vi "A170316-11_config.vi"() -> ()   [LabVIEW 2020]
uses:
  Global_Variable/Global.vi
  Database/Global1.vi
  <vilib>/Utility/config.llb/NI_LVConfig.lvlib
panel:
  in  "选项卡控件":enum32{"产品参数", "操作步骤", "产品管理"}(tab)
  in  "参数设定":string[][](table)
  in  "删除":bool
  in  "确定":bool
  in  "添加":bool
  in  "退出":bool
  in  "更新":bool
  in  "产品型号":string(combo)
  in  "安装电机操作步骤":T1
  in  "手柄安装步骤":T2
  in  "支架操作步骤":T3
  in  "请输入添加的产品名称":string
  in  "请选择要删除的产品":string(combo)
  # "调节机构装配"
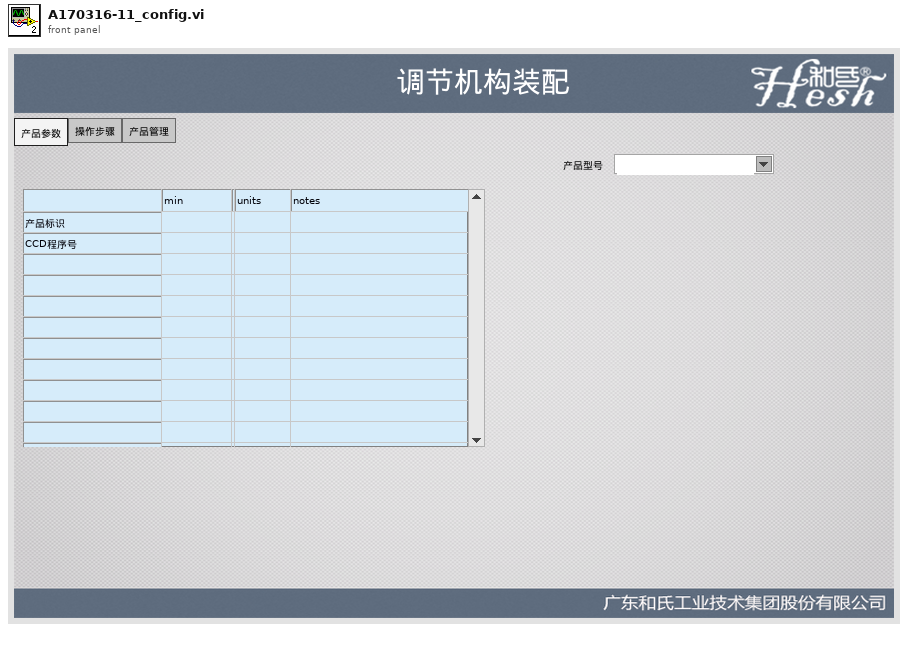
[diagram p1: front panel]
types:
  T1 = cluster{"安装弹簧":bool, "安装O型圈":bool, "安装弹性垫圈弹簧":bool, "电机安装螺栓1":bool, "电机安装螺栓2":bool, "电机安装螺栓3":bool, "电机拍照":bool, "涂色标":bool, "安装轧带":bool, "安装轧带取走工件":bool}
  T2 = cluster{"降噪垫片1/衬套1":bool, "降噪垫片2/衬套2":bool, "降噪块1":bool, "降噪块2":bool, "锁紧块":bool, "弹簧":bool, "滚针轴承":bool, "挡片":bool, "锁紧螺母":bool, "拍照":bool}
  T3 = cluster{"控制器支架螺栓1":bool, "控制器支架螺栓2":bool, "控制器支架螺栓3":bool, "控制器支架螺栓4":bool, "控制器支架螺栓5":bool, "控制器支架涂色标":bool, "控制器支架安装线束轧带":bool}
  T4 = typedef "NI_LVConfig.lvlib/Config Data RefNum.ctl" = refnum<k1>
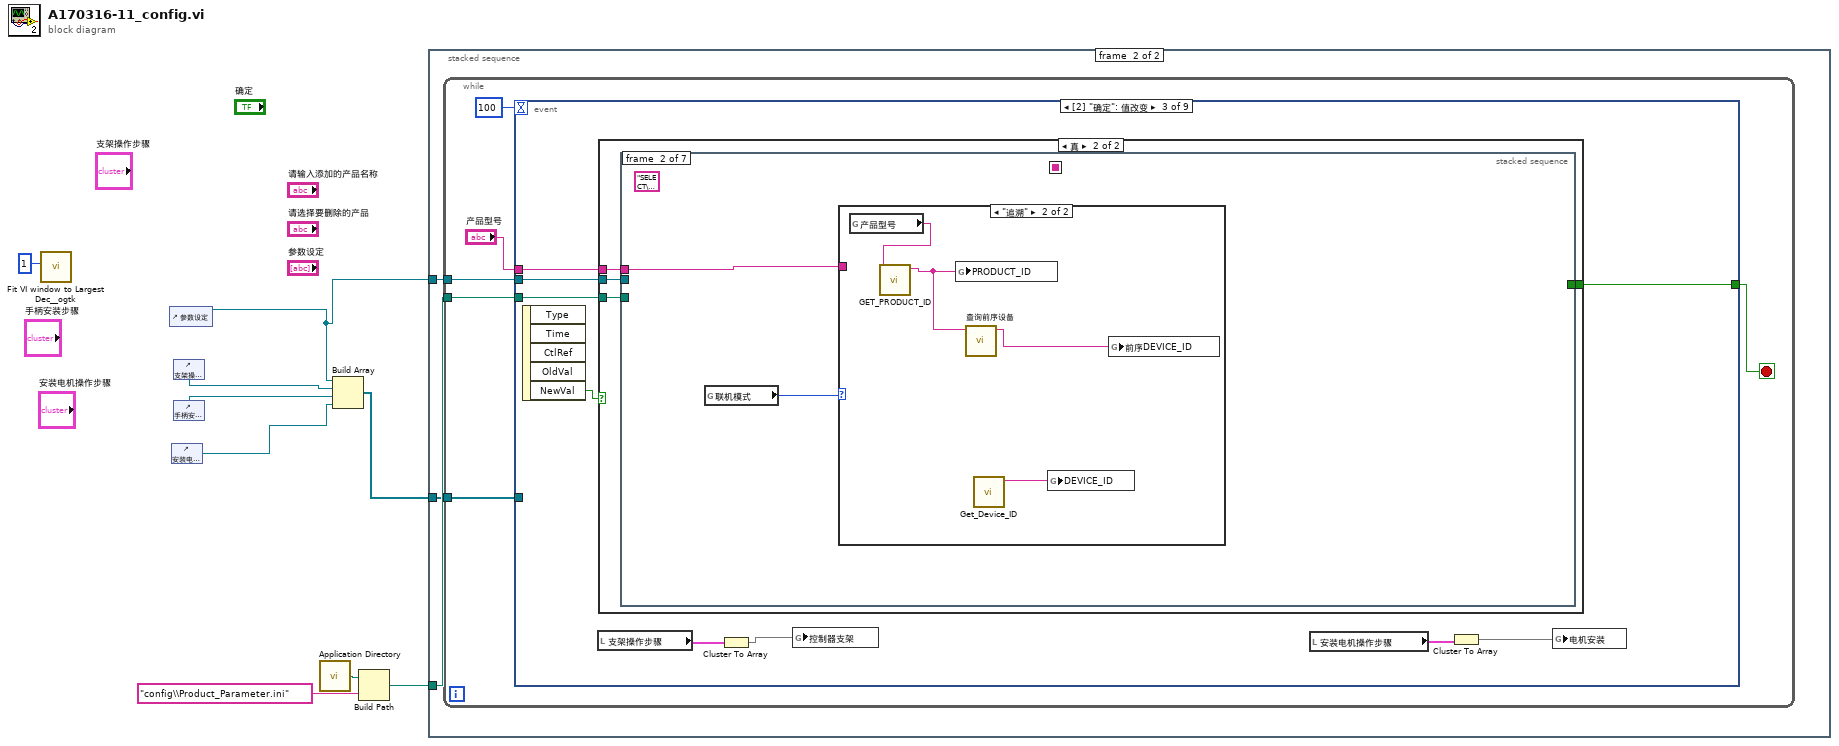
[diagram p0: block diagram]
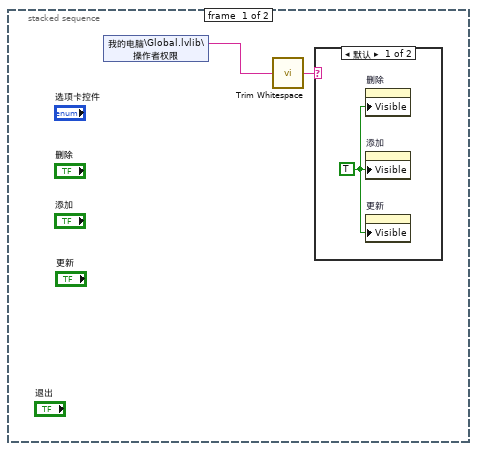
[diagram p2: hidden frame]
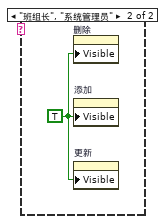
[diagram p3: hidden frame]
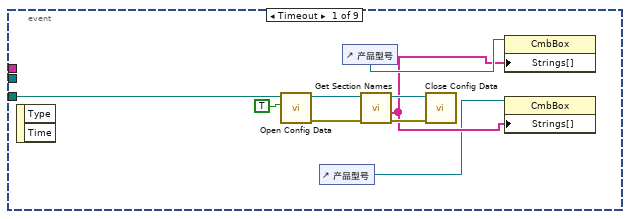
[diagram p4: hidden frame]
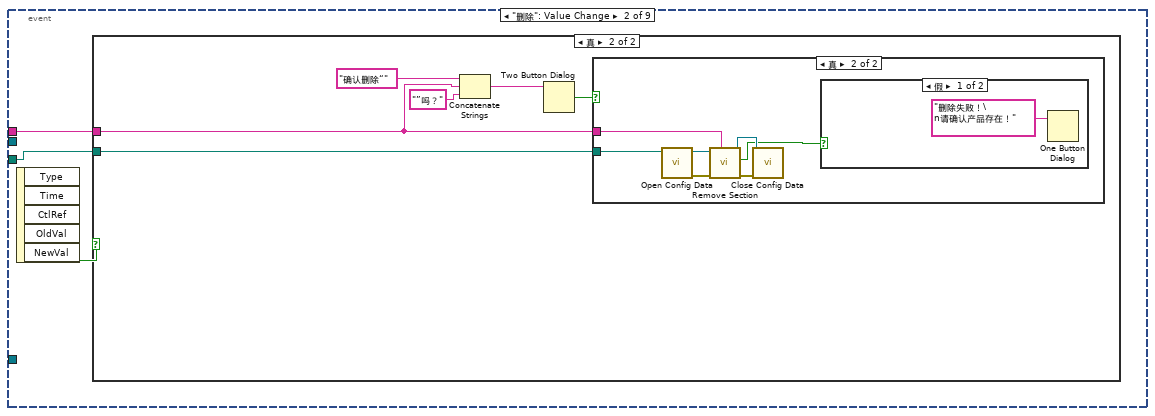
[diagram p5: hidden frame]
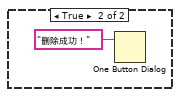
[diagram p8: hidden frame]
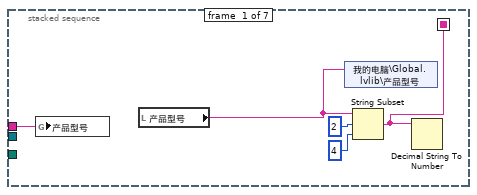
[diagram p10: hidden frame]
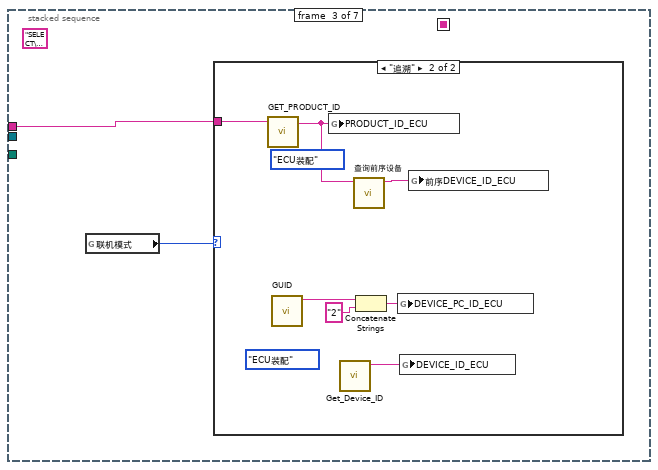
[diagram p12: hidden frame]
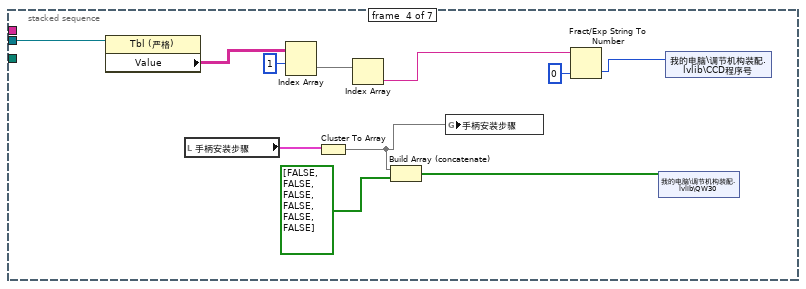
[diagram p14: hidden frame]
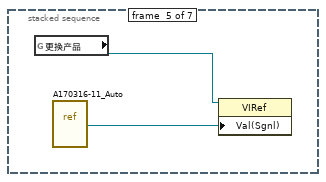
[diagram p15: hidden frame]
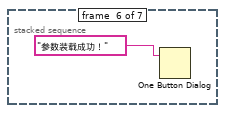
[diagram p16: hidden frame]
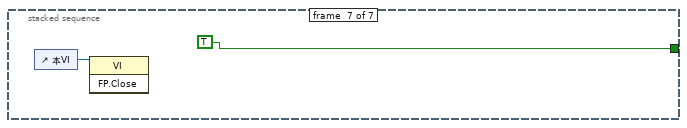
[diagram p17: hidden frame]
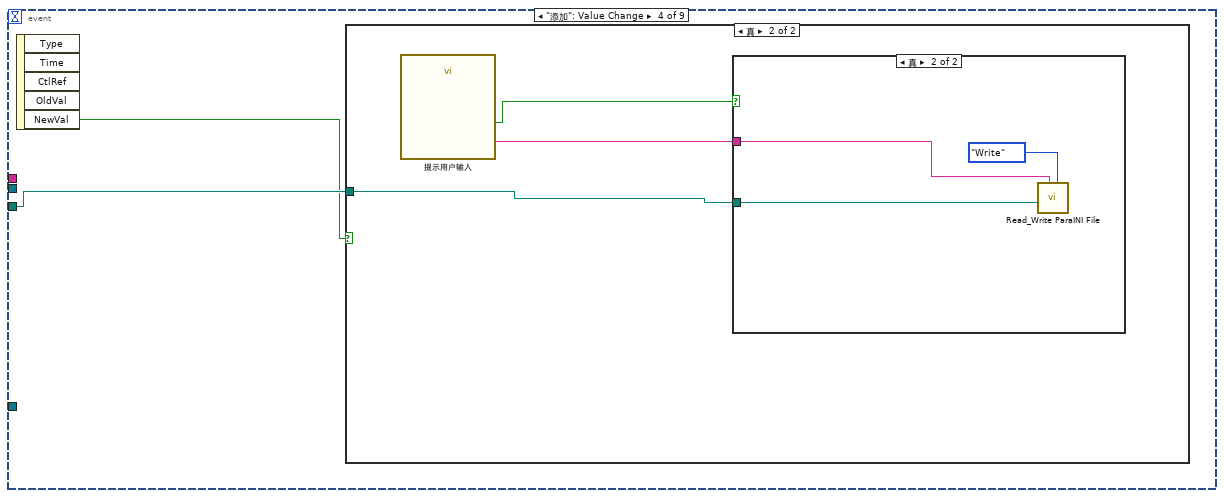
[diagram p18: hidden frame]
diagram:
  n1 = call <userlib>:"Fit VI window to Largest Dec__ogtk.vi"("border spacing (2 px)"=1) -> ()  [unwired: 5 in, 2 out]
  n2 = control-ref of="参数设定"() -> (w1:refnum<vi>)
  n3 = control-ref of="安装电机操作步骤"() -> (w3:refnum<vi>)
  n4 = control-ref of="支架操作步骤"() -> (w5:refnum<vi>)
  n5 = control-ref of="手柄安装步骤"() -> (w4:refnum<vi>)
  n6 = call <vilib>:"Application Directory.vi"() -> ("Application Directory"=w9:path)
  n7 = Build Array(w1, w5, w4, w3) -> (w2:refnum<vi>[])
  n8 = Build Path(base path=w9, name or relative path="config\\Product_Parameter.ini" ("名称或相对路径")) -> (appended path=w7:path)
  n9 = stacked-sequence {
    tunnel: w7 -> [_ w16]
    tunnel: w2 -> [_ w15]
    tunnel: w1 -> [_ w14]
    frame #0 {
      n10 = shared-variable "我的电脑\\Global.lvlib\\操作者权限"() -> (w11:string)  [unwired: 1 in, 1 out]
      n11 = call <vilib>:"Trim Whitespace.vi"("string"=w11) -> ("trimmed string"=w10:string)  [unwired: 1 in]
      n12 = case shown="默认" w10 {
        frame Default {
          w12 = TRUE ("可见")
          n13 = property on="删除" class="Bool (严格)"("Visible"=w12) -> ()  [unwired: 2 in, 2 out]
          n14 = property on="添加" class="Bool (严格)"("Visible"=w12) -> ()  [unwired: 2 in, 2 out]
          n15 = property on="更新" class="Bool (严格)"("Visible"=w12) -> ()  [unwired: 2 in, 2 out]
        }
        frame "班组长", "系统管理员" {
          w13 = TRUE ("可见")
          n16 = property on="删除" class="Bool (严格)"("Visible"=w13) -> ()  [unwired: 2 in, 2 out]
          n17 = property on="添加" class="Bool (严格)"("Visible"=w13) -> ()  [unwired: 2 in, 2 out]
          n18 = property on="更新" class="Bool (严格)"("Visible"=w13) -> ()  [unwired: 2 in, 2 out]
        }
      }
    }
    frame #1 {
      n19 = while {
        tunnel: w16 -> [w22]
        tunnel: w15 -> [w18]
        tunnel: w14 -> [w17]
        stop <- w21 stop-if-true
        n20 = event shown="[2] \"确定\": 值改变" {
          selector: _ -> [_ _ _ _ _ _ _ _ _]
          dyn-events: _ -> [_ _ _ _ _ _ _ _ _]
          timeout: 100 -> [_ _ _ _ _ _ _ _ _]
          tunnel: w22 -> [w26 w34 w56 w100 w110 _ w126 _ _]
          tunnel: [_ _ w57 _ _ TRUE _ _ TRUE] -> w21
          tunnel: "产品型号" -> [_ w32 w55 _ _ _ _ _ _]
          tunnel: w18 -> [_ _ _ _ w107 _ w124 _ _]
          tunnel: w17 -> [_ _ w50 _ _ _ _ _ _]
          event Timeout {
            n21 = event-data() -> ()  [unwired: 1 in, 2 out]
            n22 = call <vilib>:"Open Config Data.vi"("create file if necessary (T)"=TRUE, "configuration file path"=w26) -> ("error out"=w28:errorcluster, "refnum"=w27:T4)  [unwired: 7 in, 1 out]
            n23 = control-ref of="产品型号"() -> (w23:refnum<vi>)
            n24 = control-ref of="产品型号"() -> (w25:refnum<vi>)
            n25 = call <vilib>:"Get Section Names.vi"("error in (no error)"=w28, "refnum"=w27) -> ("error out"=w30:errorcluster, "section names"=w24:string[], "refnum out"=w29:T4)  [unwired: 7 in]
            n26 = call <vilib>:"Close Config Data.vi"("error in (no error)"=w30, "refnum"=w29) -> ()  [unwired: 8 in, 2 out]
            n27 = property on="属性节点" class="CmbBox"(reference=w25, "Strings[]"=w24) -> ()  [unwired: 1 in, 2 out]
            n28 = property on="属性节点" class="CmbBox"(reference=w23, "Strings[]"=w24) -> ()  [unwired: 1 in, 2 out]
          }
          event "删除": Value Change {
            n29 = event-data() -> ("NewVal"=w33:bool)  [unwired: 1 in, 4 out]
            n30 = case shown="真" w33 {
              tunnel: w34 -> [_ w36]
              tunnel: w32 -> [_ w35]
              frame False {
              }
              frame True {
                n31 = Concatenate Strings("确认删除“", w35, "”吗？") -> (w38:string)
                n32 = Two Button Dialog(message=w38) -> (T button?=w37:bool)  [unwired: 2 in]
                n33 = case shown="真" w37 {
                  tunnel: w36 -> [_ w42]
                  tunnel: w35 -> [_ w41]
                  frame False {
                  }
                  frame True {
                    n34 = call <vilib>:"Open Config Data.vi"("configuration file path"=w42) -> ("error out"=w44:errorcluster, "refnum"=w47:T4)  [unwired: 8 in, 1 out]
                    n35 = call <vilib>:"Remove Section.vi"("section"=w41, "error in (no error)"=w44, "refnum"=w47) -> ("error out"=w46:errorcluster, "section exists?"=w43:bool, "refnum out"=w45:T4)  [unwired: 6 in]
                    n36 = call <vilib>:"Close Config Data.vi"("error in (no error)"=w46, "refnum"=w45) -> ()  [unwired: 8 in, 2 out]
                    n37 = case shown="假" w43 {
                      frame False {
                        n38 = One Button Dialog(message="删除失败！\n请确认产品存在！" ("消息")) -> ()  [unwired: 1 in, 1 out]
                      }
                      frame True {
                        n39 = One Button Dialog(message="删除成功！" ("消息")) -> ()  [unwired: 1 in, 1 out]
                      }
                    }
                  }
                }
              }
            }
          }
          event "确定": Value Change {
            n40 = event-data() -> ("NewVal"=w58:bool)  [unwired: 1 in, 4 out]
            n41 = local read "支架操作步骤"() -> (w54:T3)
            n42 = case shown="真" w58 {
              tunnel: [_ w62] -> w57
              tunnel: w56 -> [_ w61]
              tunnel: w55 -> [_ w60]
              tunnel: w50 -> [_ w59]
              frame False {
              }
              frame True {
                n43 = stacked-sequence {
                  seq-local: [w67 _ _ _ _ _ _] -> [_ _ _ _ _ _ _]
                  tunnel: [_ _ _ _ _ _ TRUE] -> w62
                  tunnel: w61 -> [_ _ _ _ _ _ _]
                  tunnel: w60 -> [w66 w69 w75 _ _ _ _]
                  tunnel: w59 -> [_ _ _ w85 _ _ _]
                  frame #0 {
                    n44 = global write "Global.vi" "产品型号"(w66) -> ()
                    n45 = local read "产品型号"() -> (w65:string)
                    n46 = shared-variable "我的电脑\\Global.lvlib\\产品型号"(w65) -> ()  [unwired: 1 in, 1 out]
                    n47 = String Subset(string=w65, offset (0)=u16 2 ("偏移量(0)"), length (rest)=u16 4 ("长度（剩余）")) -> (substring=w67:string)
                    n48 = Decimal String To Number ("十进制数字符串至数值转换")(string=w67) -> ()  [unwired: 2 in, 2 out]
                  }
                  frame #1 {
                    (unwired) "SELECT\ndbo.[Product].USER_ID\nFROM\ndbo.[Product]\nWHERE\ndbo.[Product].PRODUCT_NAME = '%s'" ("格式字符串")
                    n49 = global read "Global1.vi" "联机模式"() -> (w68:enum16{"单机", "追溯"})
                    n50 = case shown="\"追溯\"" w68 {
                      tunnel: w69 -> [_ _]
                      frame "单机", Default {
                      }
                      frame "追溯" {
                        n51 = global read "Global.vi" "产品型号"() -> (w70:string)
                        n52 = call "GET_PRODUCT_ID.vi"("PRODFUCT_NAME"=w70) -> ("PRODUCT_ID"=w73:string)  [unwired: 10 in]
                        n53 = global write "Global1.vi" "PRODUCT_ID"(w73) -> ()
                        n54 = call "查询前序设备.vi"("PRODUCT_ID"=w73) -> ("前序工位"=w71:string)  [unwired: 10 in]
                        n55 = call "Get_Device_ID.vi"() -> ("Device_ID"=w72:string)  [unwired: 10 in, 1 out]
                        n56 = global write "Global1.vi" "DEVICE_ID"(w72) -> ()
                        n57 = global write "Global1.vi" "前序DEVICE_ID"(w71) -> ()
                      }
                    }
                  }
                  frame #2 {
                    (unwired) "SELECT\ndbo.[Product].USER_ID\nFROM\ndbo.[Product]\nWHERE\ndbo.[Product].PRODUCT_NAME = '%s'" ("格式字符串")
                    n58 = global read "Global1.vi" "联机模式"() -> (w74:enum16{"单机", "追溯"})
                    n59 = case shown="\"追溯\"" w74 {
                      tunnel: w75 -> [_ w81]
                      frame "单机", Default {
                      }
                      frame "追溯" {
                        (unwired) enum16{"电机装配", "ECU装配"}."ECU装配" ("枚举")
                        (unwired) enum16{"电机装配", "ECU装配"}."ECU装配" ("枚举")
                        n60 = call "GET_PRODUCT_ID.vi"("PRODFUCT_NAME"=w81) -> ("PRODUCT_ID"=w80:string)  [unwired: 10 in]
                        n61 = call "GUID.vi"() -> ("trimmed string"=w82:string)  [unwired: 11 in]
                        n62 = global write "Global1.vi" "PRODUCT_ID_ECU"(w80) -> ()
                        n63 = call "Get_Device_ID.vi"() -> ("Device_ID"=w79:string)  [unwired: 10 in, 1 out]
                        n64 = call "查询前序设备.vi"("PRODUCT_ID"=w80) -> ("前序工位"=w76:string)  [unwired: 10 in]
                        n65 = Concatenate Strings(w82, "2" ("字符串")) -> (w78:string)
                        n66 = global write "Global1.vi" "DEVICE_PC_ID_ECU"(w78) -> ()
                        n67 = global write "Global1.vi" "DEVICE_ID_ECU"(w79) -> ()
                        n68 = global write "Global1.vi" "前序DEVICE_ID_ECU"(w76) -> ()
                      }
                    }
                  }
                  frame #3 {
                    n69 = property class="Tbl (严格)"(reference=w85) -> ("Value"=w93:string[][])  [unwired: 1 in, 2 out]
                    n70 = local read "手柄安装步骤"() -> (w88:T2)
                    n71 = Index Array(array=w93, index (row)=1 ("索引 (行)")) -> (element=w91:string[])  [unwired: 1 in]
                    n72 = Cluster To Array(cluster=w88) -> (array=w86:bool[])
                    n73 = Index Array(array=w91) -> (element=w90:string)  [unwired: 1 in]
                    n74 = Build Array (concatenate)(w86, bool[] [FALSE, FALSE, FALSE, FALSE, FALSE, FALSE] ("数组")) -> (w83:bool[])
                    n75 = global write "Global.vi" "手柄安装步骤"(w86) -> ()
                    n76 = Fract/Exp String To Number(string=w90, default (0 dbl)=0 ("默认(0 DBL)")) -> (number=w84:i32)  [unwired: 2 in, 1 out]
                    n77 = shared-variable "我的电脑\\调节机构装配.lvlib\\QW30"(w83) -> ()  [unwired: 1 in, 1 out]
                    n78 = shared-variable "我的电脑\\调节机构装配.lvlib\\CCD程序号"(w84) -> ()  [unwired: 1 in, 1 out]
                  }
                  frame #4 {
                    n79 = global read "Global.vi" "更换产品"() -> (w95:refnum<vi>)
                    n80 = vi-ref "A170316-11_Auto.vi"() -> (w94:refnum<vi>)
                    n81 = property class="VIRef"(reference=w95, "Val(Sgnl)"=w94) -> ()  [unwired: 1 in, 2 out]
                  }
                  frame #5 {
                    n82 = One Button Dialog(message="参数装载成功！" ("消息")) -> ()  [unwired: 1 in, 1 out]
                  }
                  frame #6 {
                    n83 = control-ref of="本VI"() -> (w97:refnum<vi>)
                    n84 = invoke class="VI" method="FP.Close"(reference=w97) -> ()  [unwired: 2 in, 3 out]
                  }
                }
              }
            }
            n85 = Cluster To Array(cluster=w54) -> (array=w51:bool[])
            n86 = global write "Global.vi" "控制器支架"(w51) -> ()
            n87 = local read "安装电机操作步骤"() -> (w53:T1)
            n88 = Cluster To Array(cluster=w53) -> (array=w52:bool[])
            n89 = global write "Global.vi" "电机安装"(w52) -> ()
          }
          event "添加": Value Change {
            n90 = event-data() -> ("NewVal"=w99:bool)  [unwired: 1 in, 4 out]
            n91 = case shown="真" w99 {
              tunnel: w100 -> [_ w103]
              frame False {
              }
              frame True {
                n92 = call "提示用户输入"() -> ("请输入产品型号"=w102:string, "确定"=w101:bool)  [unwired: 17 in, 1 out]
                n93 = case shown="真" w101 {
                  tunnel: w103 -> [_ w106]
                  tunnel: w102 -> [_ w105]
                  frame False {
                  }
                  frame True {
                    n94 = call "Read_Write ParaINI File.vi"("Mode"=enum16{"Read", "Write"}."Write", "Section"=w105, "Filepath"=w106) -> ()  [unwired: 8 in, 1 out]
                  }
                }
              }
            }
          }
          event "产品型号": Value Change {
            n95 = event-data() -> ("CtlRef"=w109:refnum<vi>, "NewVal"=w108:string)  [unwired: 1 in, 3 out]
            n96 = stacked-sequence {
              tunnel: w110 -> [_ w118]
              tunnel: w109 -> [w112 _]
              tunnel: w108 -> [w111 _]
              tunnel: w107 -> [_ w119]
              frame #0 {
                n97 = stacked-sequence {
                  tunnel: w112 -> [_ w114]
                  tunnel: w111 -> [_ w115]
                  frame #0 {
                    n98 = control-ref of="This VI"() -> (w113:refnum<vi>)
                    n99 = invoke class="VI" method="Default Vals.Reinit All"(reference=w113) -> ()  [unwired: 2 in, 3 out]
                  }
                  frame #1 {
                    n100 = property class="CmbBox"(reference=w114, "Value"=w115) -> ()  [unwired: 1 in, 2 out]
                  }
                }
              }
              frame #1 {
                n101 = local read "产品型号"() -> (w117:string)
                n102 = call "Read_Write INI File.vi"("Mode"=enum16{"Read", "Write"}."Read", "Section"=w117, "Filepath"=w118, "Ctl Refnum"=w119) -> ()  [unwired: 7 in, 1 out]
              }
            }
          }
          event "退出": Value Change {
            n103 = event-data() -> ()  [unwired: 1 in, 5 out]
            n104 = control-ref of="本VI"() -> (w122:refnum<vi>)
            n105 = invoke class="VI" method="FP.Close"(reference=w122) -> (reference out=w120:refnum<vi>, error out=w121:errorcluster)  [unwired: 2 in, 1 out]
            n106 = Close Reference(reference=w120, error in (no error)=w121) -> ()  [unwired: 1 out]
          }
          event "更新": Value Change {
            n107 = event-data() -> ("NewVal"=w125:bool)  [unwired: 1 in, 4 out]
            n108 = case shown="真" w125 {
              tunnel: w126 -> [_ w127]
              tunnel: w124 -> [_ w128]
              frame False {
              }
              frame True {
                n109 = for {
                  tunnel: w128 -> [w133] mode=indexing
                  tunnel: w127 -> [w132]
                  n110 = local read "产品型号"() -> (w134:string)
                  n111 = call "Read_Write ParaINI File.vi"("Mode"=enum16{"Read", "Write"}."Write", "Section"=w134, "Filepath"=w132, "Ctl Refnum"=w133) -> ()  [unwired: 7 in, 1 out]
                }
                n112 = local read "产品型号"() -> (w130:string)
                n113 = call "Read_Write ParaINI File.vi"("Mode"=enum16{"Read", "Write"}."Write", "Section"=w130, "Filepath"=w127) -> ("error out"=w131:errorcluster)  [unwired: 8 in]
                n114 = case shown="无错误" w131 {
                  frame No Error {
                    n115 = call "浮动通知.vi"("通知内容"="更新成功！") -> ()  [unwired: 11 in]
                  }
                  frame Error {
                    n116 = call "浮动通知.vi"("通知内容"="更新失败！") -> ()  [unwired: 11 in]
                  }
                }
              }
            }
          }
          event "请输入添加的产品名称": Value Change {
            n117 = event-data() -> ("OldVal"=w140:string)  [unwired: 1 in, 5 out]
            n118 = control-ref of="产品型号"() -> (w138:refnum<vi>)
            n119 = property on="属性节点" class="CmbBox"(reference=w138) -> ("Strings[]"=w139:string[])  [unwired: 1 in, 2 out]
            n120 = for {
              tunnel: w140 -> [w141]
              tunnel: w139 -> [w142] mode=indexing
              n121 = Equal?(x=w141, y=w142) -> (x = y?=w143:bool)
              n122 = case shown="假" w143 {
                tunnel: w141 -> [_ w144]
                frame False {
                }
                frame True {
                  n123 = stacked-sequence {
                    tunnel: w144 -> [w150 _]
                    frame #0 {
                      w145 = 64 items=["None"=0, "Hand, Error, Stop"=16, "Question"=32, "Exclamation, Warning"=48, "Asterisk, Information"=64] ("icon")
                      w146 = 0 items=["OK", "OKCancel", "AbortRetryIgnore", "YesNoCancel", "YesNo", "RetryCancel"] ("buttons")
                      n124 = Concatenate Strings("已经存在产品”" ("text"), w150, "“\n请勿重复添加！" ("字符串")) -> (w148:string)
                      n125 = call "信息框（标题、文本、图标）.vi"("icon"=w145, "buttons"=w146, "caption"="产品重复", "text"=w148) -> ()  [unwired: 6 in, 2 out]
                    }
                    frame #1 {
                      n126 = local write "请输入添加的产品名称"("" ("请输入添加的产品名称")) -> ()
                    }
                  }
                }
              }
            }
          }
          event Panel Close {
            n127 = event-data() -> ()  [unwired: 1 in, 3 out]
          }
        }
      }
    }
  }
